vi "Untitled 2.vi"(7 "DMA Manager":refnum<class "DMA Manager.lvclass">, 8 "error in (no error)":errorcluster, 10 "Data In":refnum<data-value>) -> (0 "error out":errorcluster, 2 "Data Out":refnum<data-value>, 3 "Array out":refnum<class "1D Array s16.lvclass">)   [LabVIEW 2025]
doc: "Upload arrays from DMA enabled EDVRs to the GPU.\nFor optimal performance run this in a seperate thread (while loop) from your GPU processing loop.\nUsage of the DMA Manager is optional but can improve overal performance."
uses:
  <vilib>/Natan Biesmans/G2CPU GPU and CPU HPC Toolkit/G2CPU Libraries/Arrays/1DArray/s16/1D Array s16.lvclass
  <vilib>/Natan Biesmans/G2CPU GPU and CPU HPC Toolkit/G2CPU Libraries/Async IO/DMA Manager/DMA Manager.lvclass
  <vilib>/Natan Biesmans/G2CPU GPU and CPU HPC Toolkit/ArrayFire Driver/TypeDefs/backend.ctl
  <vilib>/Natan Biesmans/G2CPU GPU and CPU HPC Toolkit/G2CPU Libraries/Async IO/CUDA Context FGV States.ctl
  <vilib>/Natan Biesmans/G2CPU GPU and CPU HPC Toolkit/ArrayFire Driver/TypeDefs/Library Execution.ctl
  <vilib>/Natan Biesmans/G2CPU GPU and CPU HPC Toolkit/G2CPU Libraries/Arrays/Array/Array Prototype.lvclass
  <vilib>/Natan Biesmans/G2CPU GPU and CPU HPC Toolkit/ArrayFire Driver/TypeDefs/Dim4.ctl
  bc198a8f-250c-4fb0-95cf-f9e16e559b40.vi
  7a05502d-9b60-4566-9fcf-b3fb4dbedfc8.vi
  67bb9abe-6be7-467c-be3d-dc59a1f5a88b.vi
  7a05502d-9b60-4566-9fcf-b3fb4dbedfc8.vi/1a23f98f-393f-4176-8983-7f1ab824c539.vi
  <vilib>/Utility/error.llb/Error Cluster From Error Code.vi
  <vilib>/Natan Biesmans/G2CPU GPU and CPU HPC Toolkit/ArrayFire Driver/VIs/copy array.vi
  <vilib>/ErrorRing/Error Ring.xnode
  <vilib>/Natan Biesmans/G2CPU GPU and CPU HPC Toolkit/G2CPU Libraries/Async IO/G2CPU Async.lvlib
  <vilib>/Natan Biesmans/G2CPU GPU and CPU HPC Toolkit/ArrayFire Driver/AF.lvlib
  <vilib>/Natan Biesmans/G2CPU GPU and CPU HPC Toolkit/G2CPU Libraries/Manage Environment/G2CPU Manage Environment.lvlib
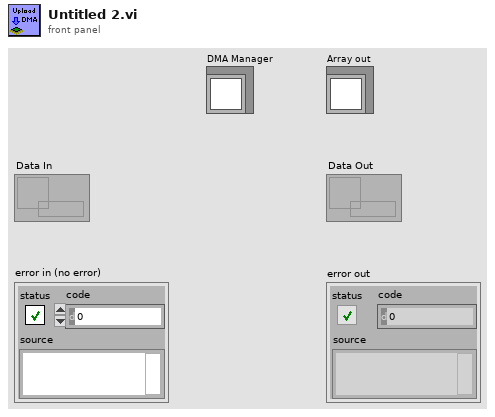
[diagram p1: front panel]
types:
  T1 = typedef "AF.lvlib/Library Execution.ctl" = enum16{"Project Settings", "Single Device", "Multi Device"}
  T2 = typedef "G2CPU Async.lvlib/CUDA Context FGV States.ctl" = enum16{"Init", "Get CUDA Context", "Release CUDA Context", "Cleanup"}
  T3 = typedef "AF.lvlib/Dim4.ctl" = cluster{"Dim 0":u64, "Dim 1":u64, "Dim 2":u64, "Dim 3":u64}
  T4 = typedef "AF.lvlib/backend.ctl" = u32
  T5 = typedef "AF.lvlib/AFType.ctl" = u32
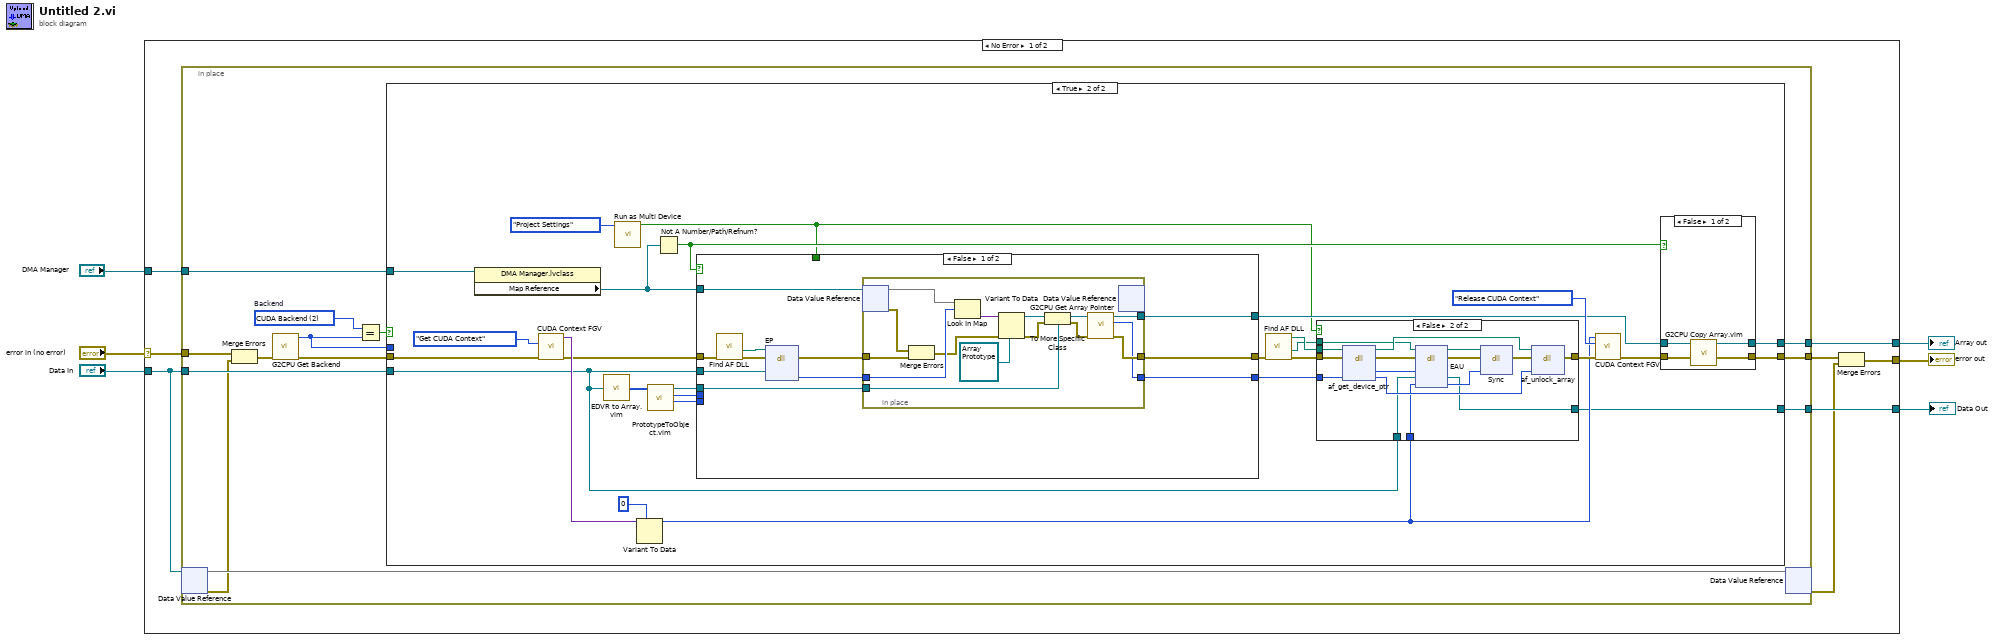
[diagram p0: block diagram]
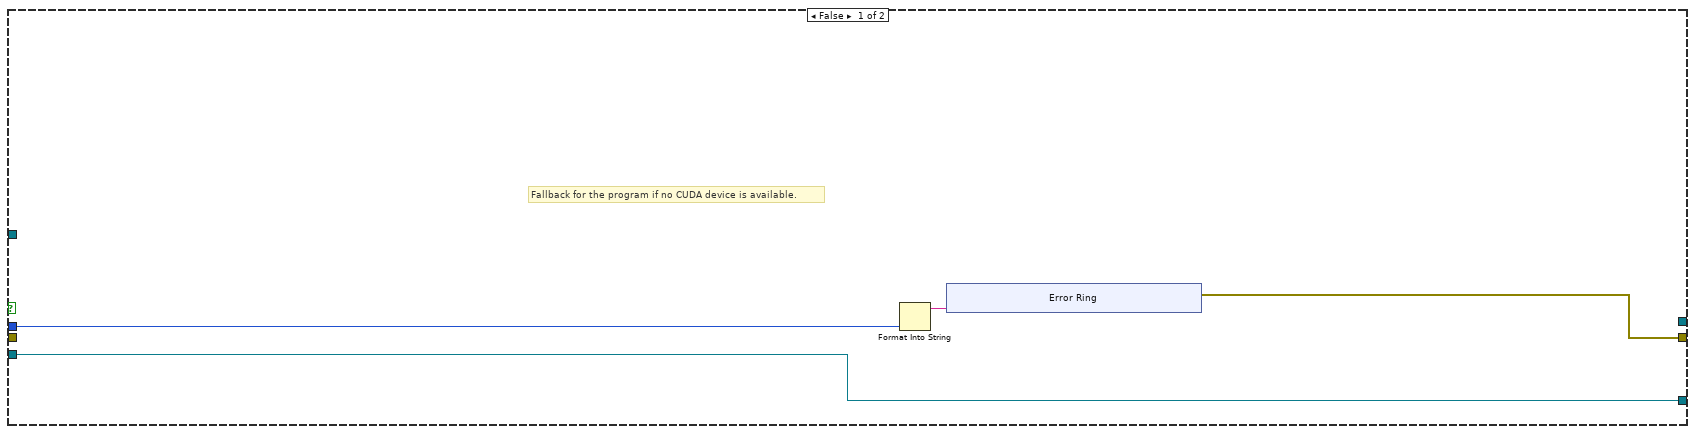
[diagram p2: hidden frame]
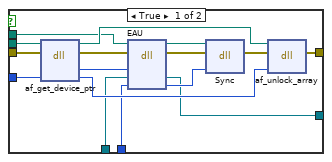
[diagram p3: hidden frame]
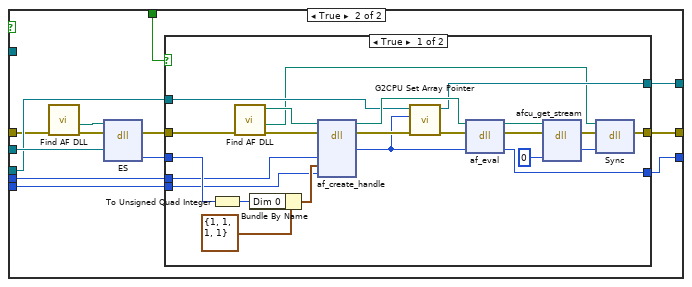
[diagram p4: hidden frame]
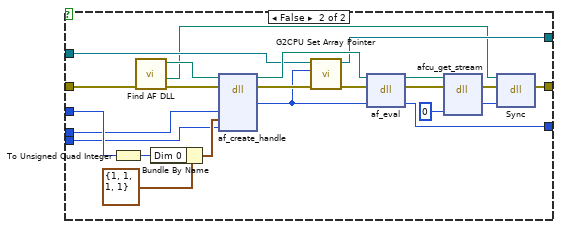
[diagram p5: hidden frame]
diagram:
  n1 = case shown="No Error" "error in (no error)" {
    selector: "error in (no error)" -> [w10 w190]
    tunnel: [w14 _] -> w6
    tunnel: [w13 _] -> w5
    tunnel: [w8 w190] -> w4
    tunnel: "DMA Manager" -> [w11 _]
    tunnel: "Data In" -> [w9 _]
    frame No Error {
      n2 = in-place {
        in-place-border: [w27] -> w14
        in-place-border: [w26] -> w13
        in-place-border: [w25] -> w12
        in-place-border: w11 -> [w24]
        in-place-border: w10 -> [w22]
        in-place-border: w9 -> [w18]
        w23 = T4 2 items=["Default Backend"=0, "CPU Backend"=1, "CUDA Backend"=2, "OPENCL Backend"=4, "Intel OneAPI Backend"=8]  # Backend
        n3 = in-place-dvr #1(w9) -> (w17:i16[], w15:errorcluster)
        n4 = Merge Errors(w22, w15) -> (w16:errorcluster)
        n5 = call <vilib>:"G2CPU Get Backend.vi"("error in (no error)"=w16) -> ("error out"=w21:errorcluster, "Backend"=w19:T4)  [unwired: 9 in]
        n6 = Equal?(x=w23, y=w19) -> (x = y?=w20:bool)
        n7 = case shown="True" w20 {
          tunnel: w21 -> [_ w58]
          tunnel: [w31 w57] -> w27
          tunnel: [_ w54] -> w26
          tunnel: [w28 w53] -> w25
          tunnel: w24 -> [_ w44]
          tunnel: w18 -> [w31 w40]
          tunnel: w19 -> [w29 _]
          frame False {
            # "Fallback for the program if no CUDA device is available."
            n8 = Format Into String(w29) -> (resulting string=w30:string)  [unwired: 3 in, 1 out]
            n9 = xnode "Error Ring"("parameter 0"=w30) -> ("error out"=w28:errorcluster)
          }
          frame True {
            n10 = property class="DMA Manager.lvclass"(reference=w44) -> ("Map Reference"=w43:refnum<data-value>)  [unwired: 1 in, 2 out]
            n11 = call <vilib>:"CUDA Context FGV.vi"("error in (no error)"=w58, "Action"=CUDA_Context_FGV_States."Get CUDA Context") -> ("error out"=w61:errorcluster, "Data out"=w65:variant)  [unwired: 8 in]
            n12 = call "EDVR to Array.vim"("CUDA Pinned Memory"=w40) -> ("Array Prototype"=w49:i16[])
            n13 = call <vilib>:"Run as Multi Device.vi"("Library Execution"=Library_Execution."Project Settings") -> ("Run as Multi Device"=w41:bool)  [unwired: 10 in]
            n14 = Variant To Data(type=u64 0 ("CudaStream"), Variant=w65) -> (data=w59:u64)  [unwired: 1 in, 1 out]
            n15 = call "PrototypeToObject.vim"("Array Prototype"=w49) -> ("type"=w46:T5, "ndims"=w47:u64, "Array Object"=w48:refnum<class "1D Array s16.lvclass">)  [unwired: 8 in]
            n16 = Not A Number/Path/Refnum?(number/path/refnum=w43) -> (NaN/Path/Refnum?=w45:bool)
            n17 = case shown="False" w45 {
              tunnel: [w109 w133] -> w62
              tunnel: w61 -> [w101 w127]
              tunnel: w43 -> [w108 _]
              tunnel: [w107 w132] -> w55
              tunnel: w40 -> [w106 w135]
              tunnel: [w105 w134] -> w52
              tunnel: w48 -> [w102 w131]
              tunnel: w47 -> [_ w130]
              tunnel: w46 -> [_ w129]
              tunnel: w41 -> [_ w128]
              frame False {
                n18 = call <vilib>:"Find AF DLL.vi"("error in (no error)"=w101) -> ("error out"=w100:errorcluster, "HS IO"=w99:path)  [unwired: 7 in, 2 out]
                n19 = dll-call lib="C:/Users/natan/Documents/G2CPU/G2CPU Libraries/Async IO/G2CPU HS IO.dll" fn="EP"(path in=w99, error in=w100, "EDVR Pointer"=w106) -> (error out=w103:errorcluster, "Ptr"=w104:i64)  [unwired: 4 in, 1 out]
                n20 = in-place {
                  in-place-border: w104 -> [w123]
                  in-place-border: [w121] -> w107
                  in-place-border: w103 -> [w120]
                  in-place-border: [w119] -> w105
                  in-place-border: [w118] -> w109
                  in-place-border: w102 -> [w110]
                  n21 = in-place-dvr #2(w108) -> (w124:map{i64, variant}, w111:errorcluster)
                  n22 = Merge Errors(w111, w120) -> (w112:errorcluster)
                  n23 = Look In Map(map=w124, key=w123) -> (value=w122:variant)  [unwired: 1 in, 1 out]
                  n24 = Variant To Data(error in=w112, type=refnum<class "Array Prototype.lvclass"> refnum ("G2CPU Arrays.lvlib:Array Prototype.lvclass"), Variant=w122) -> (data=w115:refnum<class "Array Prototype.lvclass">, error out=w114:errorcluster)
                  n25 = To More Specific Class(target class=w110, reference=w115, error in=w114) -> (specific class reference=w116:refnum<class "1D Array s16.lvclass">, error out=w113:errorcluster)
                  n26 = call <vilib>:"G2CPU Get Array Pointer.vi"("error in (no error)"=w113, "Array in"=w116) -> ("error out"=w119:errorcluster, "Array Pointer"=w118:u64, "Array out"=w121:refnum<class "1D Array s16.lvclass">)  [unwired: 7 in]
                  n27 = in-place-dvr #2() -> ()  [unwired: 1 in, 2 out]
                }
              }
              frame True {
                n28 = call <vilib>:"Find AF DLL.vi"("error in (no error)"=w127) -> ("error out"=w126:errorcluster, "HS IO"=w125:path)  [unwired: 7 in, 2 out]
                n29 = dll-call lib="C:/Users/natan/Documents/G2CPU/G2CPU Libraries/Async IO/G2CPU HS IO.dll" fn="ES"(path in=w125, error in=w126, "EDVR Pointer"=w135) -> (error out=w137:errorcluster, "Size"=w136:u32)  [unwired: 4 in, 1 out]
                n30 = case shown="True" w128 {
                  tunnel: w137 -> [w156 w179]
                  tunnel: w136 -> [w155 w178]
                  tunnel: [w144 w167] -> w134
                  tunnel: [w143 w166] -> w133
                  tunnel: [w142 w165] -> w132
                  tunnel: w131 -> [w141 w164]
                  tunnel: w130 -> [w140 w163]
                  tunnel: w129 -> [w139 w162]
                  frame True {
                    n31 = To Unsigned Quad Integer(1:w155) -> (0:w160:u64)
                    n32 = call <vilib>:"Find AF DLL.vi"("error in (no error)"=w156) -> ("error out"=w149:errorcluster, "HS IO"=w138:path, "AF Lib"=w150:path)  [unwired: 7 in, 1 out]
                    n33 = Bundle By Name(cluster=T3 {"Dim 0"=1, "Dim 1"=1, "Dim 2"=1, "Dim 3"=1} ("dims"), "Dim 0"=w160) -> (w159:T3)
                    n34 = dll-call lib="af.dll" fn="af_create_handle"(path in=w150, error in=w149, "ndims"=w140, "dims"=w159, "type"=w139) -> (path out=w151:path, error out=w158:errorcluster, "arr"=w157:u64)  [unwired: 6 in]
                    n35 = call <vilib>:"G2CPU Set Array Pointer.vi"("error in (no error)"=w158, "Array Pointer"=w157, "Array in"=w141) -> ("error out"=w152:errorcluster, "Array out"=w142:refnum<class "1D Array s16.lvclass">)  [unwired: 7 in]
                    n36 = dll-call lib="af.dll" fn="af_eval"(path in=w151, error in=w152, "Array Pointer"=w157) -> (path out=w153:path, error out=w154:errorcluster, "Array Pointer"=w143:u64)  [unwired: 2 in]
                    n37 = dll-call lib="af.dll" fn="afcu_get_stream" ("af.*:af_get_stream")(path in=w153, error in=w154, "id"=0) -> (error out=w148:errorcluster, "Stream"=w147:u64)  [unwired: 4 in, 1 out]
                    n38 = dll-call lib="C:/Users/natan/Documents/G2CPU/G2CPU Libraries/Async IO/G2CPU HS IO.dll" fn="Sync"(path in=w138, error in=w148, "CudaStream"=w147) -> (error out=w144:errorcluster)  [unwired: 3 in, 1 out]
                  }
                  frame False {
                    n39 = To Unsigned Quad Integer(1:w178) -> (0:w183:u64)
                    n40 = call <vilib>:"Find AF DLL.vi"("error in (no error)"=w179) -> ("error out"=w172:errorcluster, "HS IO"=w161:path, "AF Lib"=w173:path)  [unwired: 7 in, 1 out]
                    n41 = Bundle By Name(cluster=T3 {"Dim 0"=1, "Dim 1"=1, "Dim 2"=1, "Dim 3"=1} ("dims"), "Dim 0"=w183) -> (w182:T3)
                    n42 = dll-call lib="af.dll" fn="af_create_handle"(path in=w173, error in=w172, "ndims"=w163, "dims"=w182, "type"=w162) -> (path out=w174:path, error out=w181:errorcluster, "arr"=w180:u64)  [unwired: 6 in]
                    n43 = call <vilib>:"G2CPU Set Array Pointer.vi"("error in (no error)"=w181, "Array Pointer"=w180, "Array in"=w164) -> ("error out"=w175:errorcluster, "Array out"=w165:refnum<class "1D Array s16.lvclass">)  [unwired: 7 in]
                    n44 = dll-call lib="af.dll" fn="af_eval"(path in=w174, error in=w175, "Array Pointer"=w180) -> (path out=w176:path, error out=w177:errorcluster, "Array Pointer"=w166:u64)  [unwired: 2 in]
                    n45 = dll-call lib="af.dll" fn="afcu_get_stream" ("af.*:af_get_stream")(path in=w176, error in=w177, "id"=0) -> (error out=w171:errorcluster, "Stream"=w170:u64)  [unwired: 4 in, 1 out]
                    n46 = dll-call lib="C:/Users/natan/Documents/G2CPU/G2CPU Libraries/Async IO/G2CPU HS IO.dll" fn="Sync"(path in=w161, error in=w171, "CudaStream"=w170) -> (error out=w167:errorcluster)  [unwired: 3 in, 1 out]
                  }
                }
              }
            }
            n47 = call <vilib>:"Find AF DLL.vi"("error in (no error)"=w52) -> ("error out"=w50:errorcluster, "HS IO"=w39:path, "AF Lib"=w51:path)  [unwired: 7 in, 1 out]
            n48 = case shown="False" w41 {
              tunnel: w62 -> [w79 w95]
              tunnel: [w76 w92] -> w60
              tunnel: w59 -> [w73 w89]
              tunnel: [w72 w88] -> w57
              tunnel: w51 -> [w71 w87]
              tunnel: w50 -> [w70 w86]
              tunnel: w40 -> [w69 w85]
              tunnel: w39 -> [w68 w84]
              frame True {
                n49 = dll-call lib="af.dll" fn="af_get_device_ptr"(path in=w71, error in=w70, "Array Pointer"=w79) -> (path out=w77:path, error out=w75:errorcluster, "device Ptr"=w74:u64, "Array Pointer"=w80:u64)  [unwired: 3 in]
                n50 = dll-call lib="C:/Users/natan/Documents/G2CPU/G2CPU Libraries/Async IO/G2CPU HS IO.dll" fn="EAU"(path in=w68, error in=w75, "dst"=w74, "src"=w69, "CudaStream"=w73) -> (path out=w67:path, error out=w82:errorcluster, "src"=w72:refnum<data-value>, "CudaStream"=w81:u64)  [unwired: 3 in]
                n51 = dll-call lib="C:/Users/natan/Documents/G2CPU/G2CPU Libraries/Async IO/G2CPU HS IO.dll" fn="Sync"(path in=w67, error in=w82, "CudaStream"=w81) -> (error out=w78:errorcluster)  [unwired: 3 in, 1 out]
                n52 = dll-call lib="af.dll" fn="af_unlock_array"(path in=w77, error in=w78, "Array Pointer"=w80) -> (error out=w76:errorcluster)  [unwired: 3 in, 1 out]
              }
              frame False {
                n53 = dll-call lib="af.dll" fn="af_get_device_ptr"(path in=w87, error in=w86, "Array Pointer"=w95) -> (path out=w93:path, error out=w91:errorcluster, "device Ptr"=w90:u64, "Array Pointer"=w96:u64)  [unwired: 3 in]
                n54 = dll-call lib="C:/Users/natan/Documents/G2CPU/G2CPU Libraries/Async IO/G2CPU HS IO.dll" fn="EAU"(path in=w84, error in=w91, "dst"=w90, "src"=w85, "CudaStream"=w89) -> (path out=w83:path, error out=w98:errorcluster, "src"=w88:refnum<data-value>, "CudaStream"=w97:u64)  [unwired: 3 in]
                n55 = dll-call lib="C:/Users/natan/Documents/G2CPU/G2CPU Libraries/Async IO/G2CPU HS IO.dll" fn="Sync"(path in=w83, error in=w98, "CudaStream"=w97) -> (error out=w94:errorcluster)  [unwired: 3 in, 1 out]
                n56 = dll-call lib="af.dll" fn="af_unlock_array"(path in=w93, error in=w94, "Array Pointer"=w96) -> (error out=w92:errorcluster)  [unwired: 3 in, 1 out]
              }
            }
            n57 = call <vilib>:"CUDA Context FGV.vi"("error in (no error)"=w60, "Action"=CUDA_Context_FGV_States."Release CUDA Context", "Data in"=w59) -> ("error out"=w56:errorcluster)  [unwired: 7 in, 1 out]
            n58 = case shown="False" w45 {
              tunnel: w56 -> [w187 w188]
              tunnel: w55 -> [w186 w189]
              tunnel: [w185 w189] -> w54
              tunnel: [w184 w188] -> w53
              frame False {
                n59 = call "G2CPU Copy Array.vim"("error in (no error)"=w187, "Array In"=w186) -> ("error out"=w184:errorcluster, "Copied Array"=w185:refnum<class "1D Array s16.lvclass">)  [unwired: 8 in]
              }
              frame True {
              }
            }
          }
        }
        n60 = in-place-dvr #1(w17) -> (w7:errorcluster)  [unwired: 1 out]
      }
      n61 = Merge Errors(w12, w7) -> (w8:errorcluster)
    }
    frame Error {
    }
  }
  "error out" <- w4
  "Array out" <- w5
  "Data Out" <- w6
